vi "ex_SaveFileCheckNameTDM.vi"(4 "file exists?":bool, 5 "overwrite_mode_multi":T3(ring)=enum."overwrite & backup", 6 "multi_file":bool, 7 "overwrite_mode":T4(ring), 8 "error in (no error)":errorcluster, 10 "file params in":T1={"delimiter"="\t", "origin time"=timestamp(0 s since 1904-01-01), "Flags"={"include col headings?"=TRUE, "x_columns"=0, "col headings always?"=TRUE, "time preference"=0, "hide col headings"=FALSE}, "Decimal Separator"=""} {"Flags"."time preference" items=["Absolute", "Relative"]; "Flags"."x_columns" items=["None", "One", "Multiple"]; "origin time" format="%<%X\n%x>T"}, 11 "file path":path) -> (0 "error out":errorcluster, 1 "Storage RefNum":refnum<k20>, 2 "file params out":T1={"delimiter"="\t", "origin time"=timestamp(0 s since 1904-01-01), "Flags"={"include col headings?"=TRUE, "x_columns"=0, "col headings always?"=TRUE, "time preference"=0, "hide col headings"=FALSE}, "Decimal Separator"=""} {"Flags"."time preference" items=["Absolute", "Relative"]; "Flags"."x_columns" items=["None", "One", "Multiple"]; "origin time" format="%<%X\n%x>T"}, 3 "file path out":path)   [LabVIEW 2017]
uses:
  <vilib>/express/express output/ExFileWriteBlock.llb/ex_WriteFileParams.ctl
  <vilib>/express/express input/ExFileReadBlock.llb/ex_ReadFileParams.ctl
  <vilib>/express/express shared/ExFile.llb/ex_FileFormatSelector.ctl
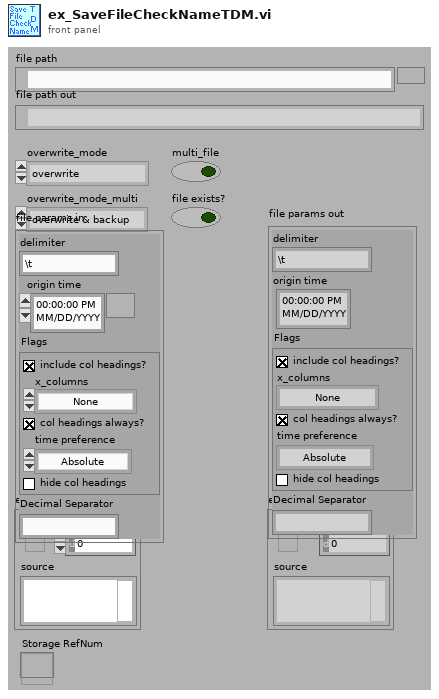
[diagram p1: front panel]
types:
  T1 = typedef "ex_WriteFileParams.ctl" = cluster{"delimiter":string, "origin time":timestamp, "Flags":T2, "Decimal Separator":string}
  T2 = typedef "ex_ReadFileParams.ctl" = cluster{"include col headings?":bool, "x_columns":u16, "col headings always?":bool, "time preference":u16, "hide col headings":bool}
  T3 = enum16{"overwrite", "overwrite & backup", "next avail"}
  T4 = enum16{"overwrite", "overwrite & backup", "append", "next avail"}
  T5 = typedef "ex_FileFormatSelector.ctl" = enum32{"lvm", "tdm", "other"}
  T6 = enum16{"open", "open or create", "create or replace", "create", "open (read only)"}
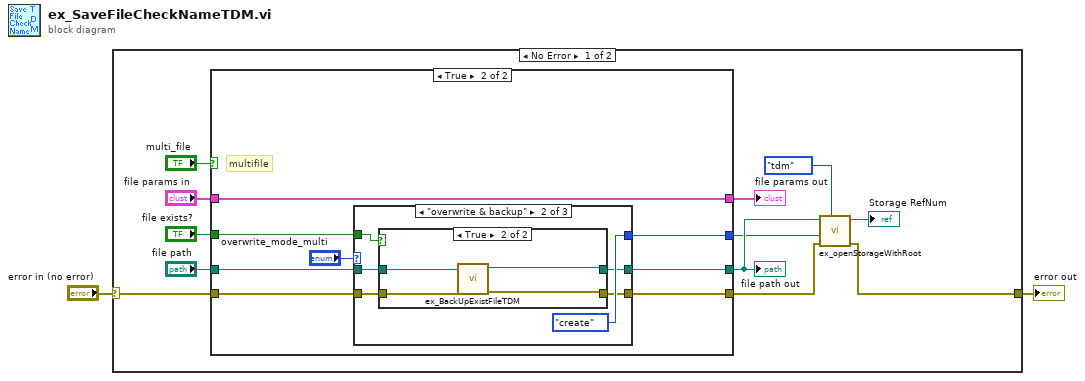
[diagram p0: block diagram]
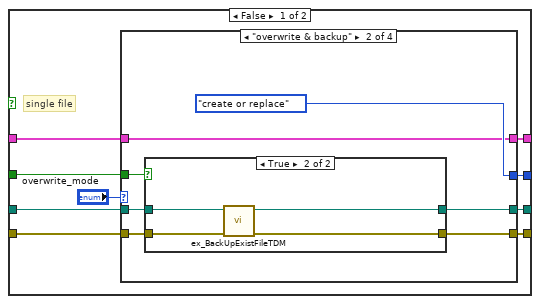
[diagram p2: hidden frame]
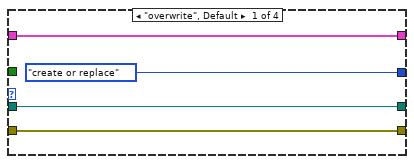
[diagram p3: hidden frame]
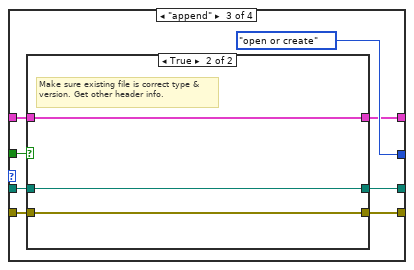
[diagram p5: hidden frame]
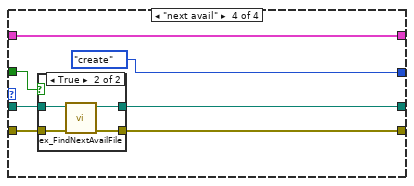
[diagram p7: hidden frame]
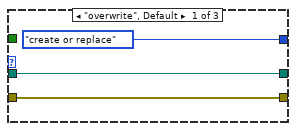
[diagram p9: hidden frame]
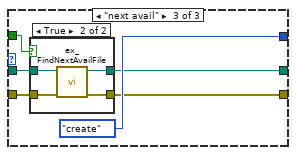
[diagram p11: hidden frame]
diagram:
  n1 = case shown="No Error" "error in (no error)" {
    selector: "error in (no error)" -> [w11 w103]
    tunnel: [w7 w103] -> w2
    frame No Error {
      n2 = case shown="True" "multi_file" {
        tunnel: [w22 w74] -> w4
        tunnel: "file path" -> [w17 w73]
        tunnel: [w19 w71] -> w6
        tunnel: [w18 w70] -> w8
        tunnel: "file exists?" -> [w21 w69]
        tunnel: w11 -> [w20 w72]
        tunnel: [w15 w68] -> w9
        tunnel: "file params in" -> [w16 w68]
        frame False {
          # "single file"
          n3 = case shown="\"overwrite & backup\"" "overwrite_mode" {
            tunnel: [T6."create or replace" ("function (open:0)") T6."create or replace" ("function (open:0)") T6."open or create" ("function (open:0)") T6."create" ("function (open:0)")] -> w22
            tunnel: w21 -> [_ w29 w46 w56]
            tunnel: w17 -> [w26 w31 w42 w60]
            tunnel: w20 -> [w25 w30 w47 w57]
            tunnel: [w26 w33 w41 w58] -> w19
            tunnel: [w25 w32 w45 w59] -> w18
            tunnel: [w24 w28 w44 w55] -> w15
            tunnel: w16 -> [w24 w28 w43 w55]
            frame "overwrite", Default {
            }
            frame "overwrite & backup" {
              n4 = case shown="True" w29 {
                tunnel: w31 -> [w35 w40]
                tunnel: w30 -> [w36 w39]
                tunnel: [w35 w37] -> w33
                tunnel: [w36 w38] -> w32
                frame False {
                  # "File doesn't exist-- do nothing"
                }
                frame True {
                  n5 = call <vilib>:"ex_BackUpExistFileTDM.vi"("error in"=w39, "file path"=w40) -> ("error out"=w38:errorcluster, "dup file path"=w37:path)  [unwired: 8 out]
                }
              }
            }
            frame "append" {
              n6 = case shown="True" w46 {
                tunnel: w47 -> [w50 w52]
                tunnel: w42 -> [w49 w54]
                tunnel: [w50 w52] -> w45
                tunnel: [w51 w53] -> w44
                tunnel: w43 -> [w51 w53]
                tunnel: [w49 w54] -> w41
                frame False {
                }
                frame True {
                  # "Make sure existing file is correct type & version. Get other header info."
                }
              }
            }
            frame "next avail" {
              n7 = case shown="True" w56 {
                tunnel: w60 -> [w63 w67]
                tunnel: [w62 w66] -> w59
                tunnel: [w63 w65] -> w58
                tunnel: w57 -> [w62 w64]
                frame False {
                }
                frame True {
                  n8 = call <vilib>:"ex_FindNextAvailFile.vi"("error in"=w64, "desired file path"=w67) -> ("error out"=w66:errorcluster, "next avail file path"=w65:path)  [unwired: 8 out]
                }
              }
            }
          }
        }
        frame True {
          # "multifile"
          n9 = case shown="\"overwrite & backup\"" "overwrite_mode_multi" {
            tunnel: [T6."create or replace" ("function (open:0)") T6."create" ("function (open:0)") T6."create" ("function (open:0)")] -> w74
            tunnel: w73 -> [w77 w83 w93]
            tunnel: w72 -> [w76 w82 w92]
            tunnel: [w77 w80 w95] -> w71
            tunnel: [w76 w79 w94] -> w70
            tunnel: w69 -> [_ w81 w91]
            frame "overwrite", Default {
            }
            frame "overwrite & backup" {
              n10 = case shown="True" w81 {
                tunnel: w83 -> [w85 w90]
                tunnel: w82 -> [w86 w89]
                tunnel: [w85 w88] -> w80
                tunnel: [w86 w87] -> w79
                frame False {
                  # "File doesn't exist-- do nothing"
                }
                frame True {
                  n11 = call <vilib>:"ex_BackUpExistFileTDM.vi"("error in"=w89, "file path"=w90) -> ("error out"=w87:errorcluster, "dup file path"=w88:path)  [unwired: 8 out]
                }
              }
            }
            frame "next avail" {
              n12 = case shown="True" w91 {
                tunnel: w93 -> [w98 w102]
                tunnel: [w97 w101] -> w94
                tunnel: [w98 w100] -> w95
                tunnel: w92 -> [w97 w99]
                frame False {
                }
                frame True {
                  n13 = call <vilib>:"ex_FindNextAvailFile.vi"("error in"=w99, "desired file path"=w102) -> ("error out"=w101:errorcluster, "next avail file path"=w100:path)  [unwired: 8 out]
                }
              }
            }
          }
        }
      }
      "file path out" <- w6
      "file params out" <- w9
      n14 = call <vilib>:"ex_openStorageWithRoot.vi"("storage_format"=ex_FileFormatSelector."tdm", "error in (no error)"=w8, "Overwrite Options"=w4, "Storage Location"=w6) -> ("error out"=w7:errorcluster, "Data Object"=→"Storage RefNum":refnum<k20>)  [unwired: 1 in, 5 out]
    }
    frame Error {
    }
  }
  "error out" <- w2
